vi "MULTTCP2_CmdHandler.vi"(0 "logfile":path, 1 "taskID":string, 2 "async on block":refnum<vi>, 3 "cmd queue":refnum<queue>, 5 "Log":bool, 7 "cmdref":refnum<vi>, 9 "respref":refnum<vi>, 10 "info cluster":T1, 11 "error cmd out":errorcluster, 12 "error resp out":errorcluster, 13 "last cmd":refnum<vi>, 14 "last response":refnum<vi>) -> (15 "error resp out":errorcluster)   [LabVIEW 2016]
uses:
  public/vis/coms/TCPSERVER/private/vis/PAN_TCPSERVER_MsgStruct.ctl
  DBSHAND/private/vis/DatabaseHand_Element_Get(string).vi
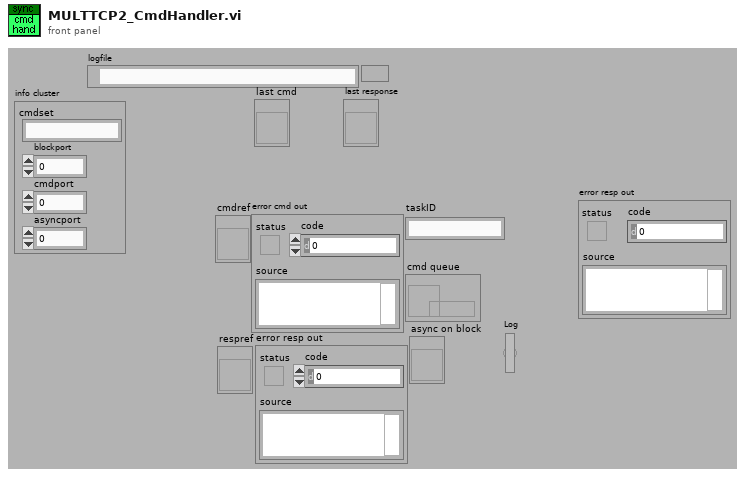
[diagram p1: front panel]
types:
  T1 = cluster{"cmdset":string, "blockport":u16, "cmdport":u16, "asyncport":u16}
  T2 = typedef "DatabaseHand_RefNum.ctl" = refnum<vi>
  T3 = typedef "PAN_TCPSERVER_MsgStruct.ctl" = cluster{"ID":string, "socket ID":refnum<k5>, "messages out queue":refnum<queue>, "message received":string, "type":string}
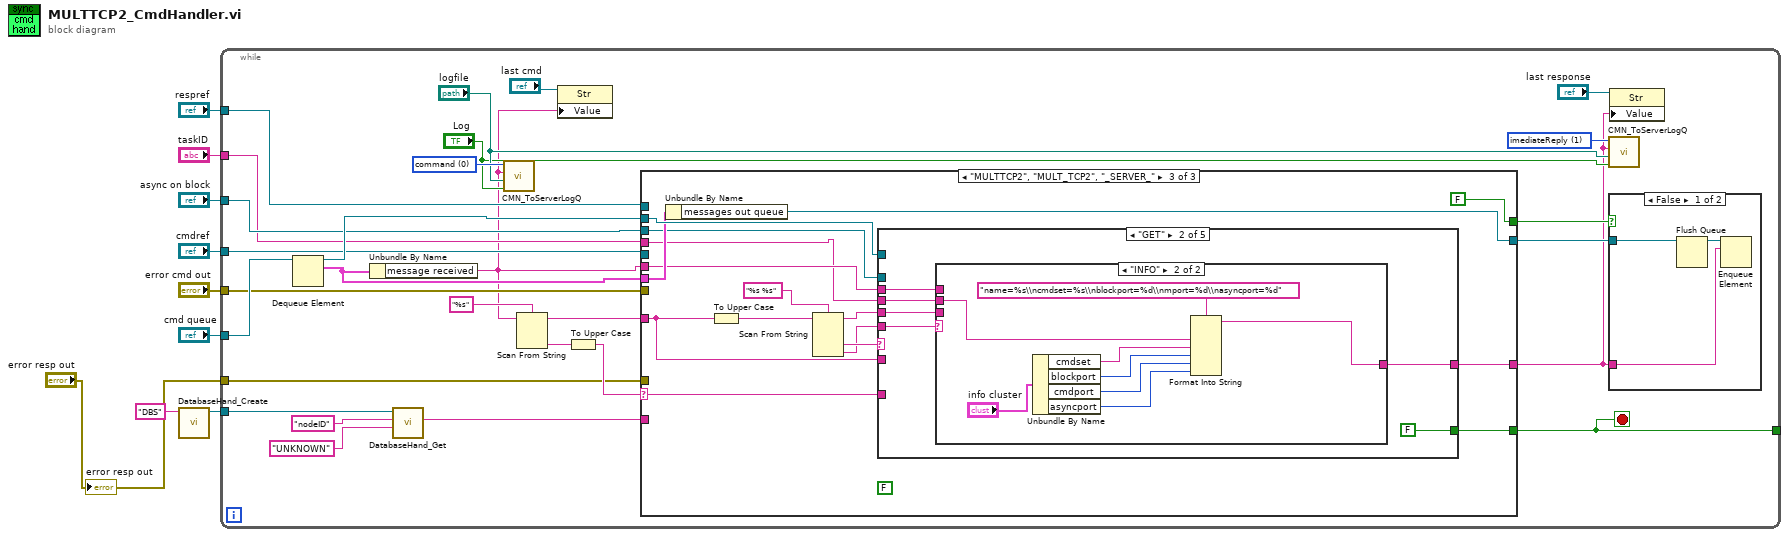
[diagram p0: block diagram]
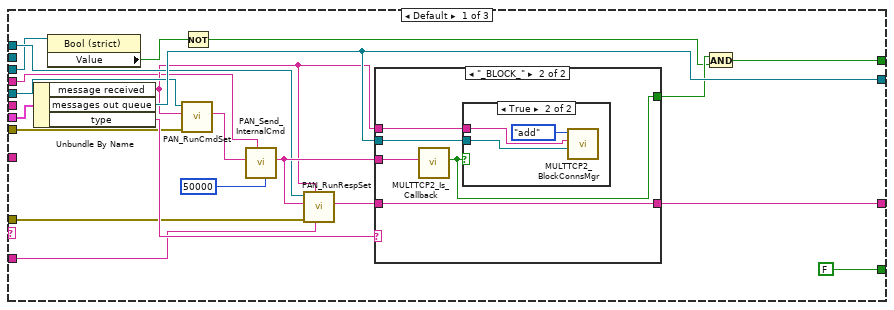
[diagram p3: hidden frame]
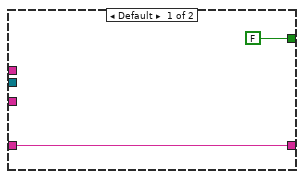
[diagram p4: hidden frame]
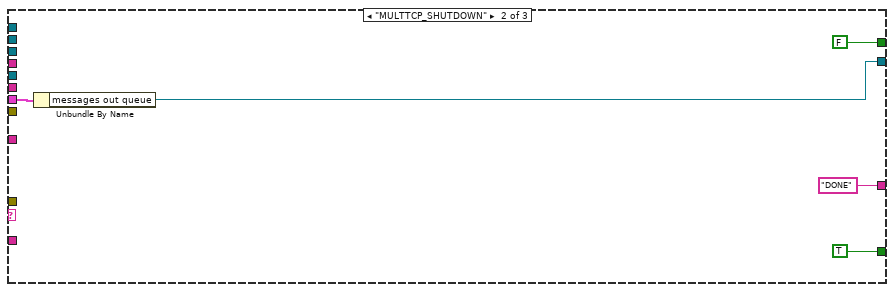
[diagram p6: hidden frame]
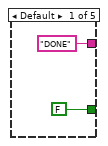
[diagram p7: hidden frame]
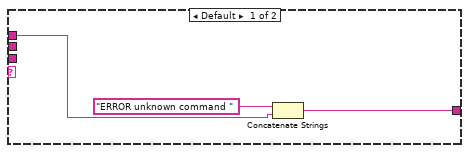
[diagram p8: hidden frame]
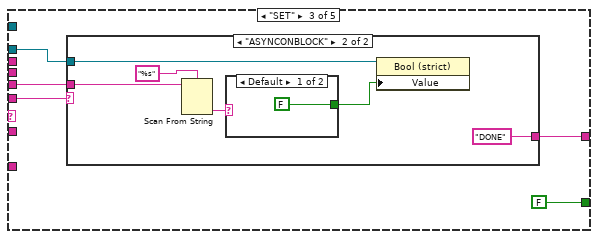
[diagram p9: hidden frame]
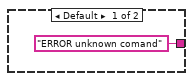
[diagram p10: hidden frame]
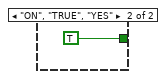
[diagram p11: hidden frame]
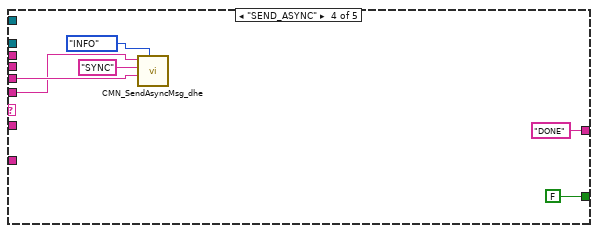
[diagram p12: hidden frame]
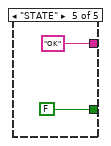
[diagram p13: hidden frame]
diagram:
  n1 = call "DatabaseHand_Create.vi"("Name"="DBS") -> ("Database RefNum out"=w8:T2)  [unwired: 1 in, 9 out]
  n2 = while {
    tunnel: "cmd queue" -> [w37]
    tunnel: [w32] -> _
    tunnel: "cmdref" -> [w25]
    tunnel: "error cmd out" -> [w24]
    tunnel: "respref" -> [w23]
    tunnel: "error resp out" -> [w22]
    tunnel: w8 -> [w20]
    tunnel: "async on block" -> [w16]
    tunnel: "taskID" -> [w15]
    stop <- w32 stop-if-true
    w26 = u16 0 items=["command", "imediateReply", "Callback Reply", "Information", "none"] ("type")
    w27 = u16 1 items=["command", "imediateReply", "Callback Reply", "Information", "none"] ("type")
    n3 = Dequeue Element(queue=w37) -> (queue out=w30:refnum<queue>, element=w34:T3)  [unwired: 1 in, 3 out]
    n4 = Unbundle By Name(w34) -> ("message received"=w13:string)
    n5 = call-poly "DatabaseHand_Get.vi"("default value"="UNKNOWN", "name"="nodeID", "Database RefNum in"=w20) -> ("value"=w19:string)  [unwired: 2 in, 6 out]
    n6 = call "CMN_ToServerLogQ.vi"("Log"="Log", "file"="logfile", "string"=w13, "type"=w26) -> ()  [unwired: 2 in, 5 out]
    n7 = Scan From String(format string="%s", input string=w13) -> (remaining string=w33:string, output 1=w31:string)  [unwired: 2 in, 3 out]
    n8 = property class="Str"(reference="last cmd", "Value"=w13) -> ()  [unwired: 1 in, 2 out]
    n9 = To Upper Case(1:w31) -> (0:w35:string)
    n10 = case shown="\"MULTTCP2\", \"MULT_TCP2\", \"_SERVER_\"" w35 {
      selector: w35 -> [_ _ w91]
      tunnel: [FALSE TRUE w92] -> w32
      tunnel: w34 -> [w61 w76 w83]
      tunnel: w33 -> [_ _ w79]
      tunnel: [w57 "DONE" ("data in") w90] -> w11
      tunnel: w30 -> [_ _ w84]
      tunnel: [w58 w72 w82] -> w29
      tunnel: [w46 FALSE ("blocking") FALSE] -> w28
      tunnel: w13 -> [_ _ w81]
      tunnel: w25 -> [w52 _ _]
      tunnel: w24 -> [w51 _ _]
      tunnel: w23 -> [w50 _ _]
      tunnel: w22 -> [w49 _ _]
      tunnel: w19 -> [w47 _ _]
      tunnel: w16 -> [w43 _ w78]
      tunnel: w15 -> [w41 _ w77]
      frame Default {
        n11 = Unbundle By Name(w61) -> ("message received"=w48:string, "messages out queue"=w58:refnum<queue>, "type"=w59:string)
        n12 = property class="Bool (strict)"(reference=w43) -> ("Value"=w42:bool)  [unwired: 1 in, 2 out]
        n13 = call "PAN_RunCmdSet.vi"("error in (no error)"=w51, "cmd in"=w48, "type specifier VI Refnum (for type only)"=w52) -> ("cmd out"=w55:string)  [unwired: 8 out]
        n14 = Not(x=w42) -> (.not. x?=w44:bool)
        n15 = call "PAN_Send_InternalCmd.vi"("timeout in ms (-1)"=50000, "taskID"=w41, "command"=w55) -> ("response"=w54:string)  [unwired: 2 in, 6 out]
        n16 = call "PAN_RunRespSet.vi"("nodeID"=w47, "cmd in"=w48, "error in (no error)"=w49, "resp in"=w54, "type specifier VI Refnum (for type only)"=w50) -> ("resp out"=w53:string)  [unwired: 6 out]
        n17 = case shown="\"_BLOCK_\"" w59 {
          tunnel: [FALSE w67] -> w45
          tunnel: w58 -> [_ w68]
          tunnel: w54 -> [_ w66]
          tunnel: [w62 w64] -> w57
          tunnel: w48 -> [_ w65]
          tunnel: w53 -> [w62 w64]
          frame Default {
          }
          frame "_BLOCK_" {
            n18 = call "MULTTCP2_Is_Callback.vi"("Connections"=w66) -> ("callback?"=w67:bool)  [unwired: 2 in, 8 out]
            n19 = case shown="True" w67 {
              tunnel: w68 -> [_ w71]
              tunnel: w65 -> [_ w69]
              frame False {
              }
              frame True {
                n20 = call "MULTTCP2_BlockConnsMgr.vi"("message back  queue"=w71, "arg"=w69, "action"=enum16{"add", "delete"}."add") -> ()  [unwired: 1 in, 8 out]
              }
            }
          }
        }
        n21 = And(x=w45, y=w44) -> (x .and. y?=w46:bool)
      }
      frame "MULTTCP_SHUTDOWN" {
        n22 = Unbundle By Name(w76) -> ("messages out queue"=w72:refnum<queue>)
      }
      frame "MULTTCP2", "MULT_TCP2", "_SERVER_" {
        (unwired) FALSE ("callback?")
        n23 = Unbundle By Name(w83) -> ("messages out queue"=w82:refnum<queue>)
        n24 = To Upper Case(1:w79) -> (0:w85:string)
        n25 = Scan From String(format string="%s %s", input string=w85) -> (remaining string=w86:string, output 1=w88:string, output 2=w87:string)  [unwired: 2 in, 4 out]
        n26 = case shown="\"GET\"" w88 {
          tunnel: [FALSE FALSE FALSE FALSE FALSE] -> w92
          tunnel: w91 -> [_ _ _ _ _]
          tunnel: ["DONE" ("data in") w98 w114 "DONE" ("data in") "OK" ("data in")] -> w90
          tunnel: w87 -> [_ w100 w116 w127 _]
          tunnel: w86 -> [_ w96 w115 w128 _]
          tunnel: w84 -> [_ _ _ _ _]
          tunnel: w81 -> [_ w97 _ _ _]
          tunnel: w79 -> [_ _ _ _ _]
          tunnel: w78 -> [_ _ w112 _ _]
          tunnel: w77 -> [_ w95 _ _ _]
          frame Default {
          }
          frame "GET" {
            n27 = case shown="\"INFO\"" w100 {
              tunnel: [w101 w104] -> w98
              tunnel: w97 -> [w102 _]
              tunnel: w96 -> [_ _]
              tunnel: w95 -> [_ w105]
              frame Default {
                n28 = Concatenate Strings("ERROR unknown command " ("response"), w102) -> (w101:string)
              }
              frame "INFO" {
                n29 = Unbundle By Name("info cluster") -> ("cmdset"=w109:string, "blockport"=w108:u16, "cmdport"=w107:u16, "asyncport"=w106:u16)
                n30 = Format Into String(format string="name=%s\\ncmdset=%s\\nblockport=%d\\nmport=%d\\nasyncport=%d", w105, w109, w108, w107, w106) -> (resulting string=w104:string)  [unwired: 2 in, 1 out]
              }
            }
          }
          frame "SET" {
            n31 = case shown="\"ASYNCONBLOCK\"" w116 {
              tunnel: w115 -> [_ w123]
              tunnel: ["ERROR unknown comand" "DONE"] -> w114
              tunnel: w112 -> [_ w118]
              frame Default {
              }
              frame "ASYNCONBLOCK" {
                n32 = Scan From String(format string="%s", input string=w123) -> (output 1=w121:string)  [unwired: 2 in, 4 out]
                n33 = case shown="Default" w121 {
                  tunnel: [FALSE ("async_on_block") TRUE ("async_on_block")] -> w120
                  frame Default {
                  }
                  frame "ON", "TRUE", "YES" {
                  }
                }
                n34 = property on="Property Node" class="Bool (strict)"(reference=w118, "Value"=w120) -> ()  [unwired: 1 in, 2 out]
              }
            }
          }
          frame "SEND_ASYNC" {
            n35 = call "CMN_SendAsyncMsg_dhe.vi"("type"=enum16{"ERROR", "WARNING", "INFO", "CHANGED"}."INFO", "Message"=w128, "device"="SYNC", "command"=w127) -> ()  [unwired: 8 out]
          }
          frame "STATE" {
          }
        }
      }
    }
    n36 = call "CMN_ToServerLogQ.vi"("Log"="Log", "file"="logfile", "string"=w11, "type"=w27) -> ()  [unwired: 2 in, 5 out]
    n37 = case shown="False" w28 {
      tunnel: w11 -> [w38 _]
      tunnel: w29 -> [w40 _]
      frame False {
        n38 = Flush Queue(queue=w40) -> (queue out=w39:refnum<queue>)  [unwired: 1 in, 2 out]
        n39 = Enqueue Element(queue=w39, element=w38) -> ()  [unwired: 1 in, 4 out]
      }
      frame True {
      }
    }
    n40 = property class="Str"(reference="last response", "Value"=w11) -> ()  [unwired: 1 in, 2 out]
  }
  "error resp out" <- "error resp out"
